vi "Data Transmit.vi"() -> ()   [LabVIEW 2021]
panel:
  in  "Message":string
  in  "Boolean":bool
  out "error out":errorcluster
  in  "error in":errorcluster
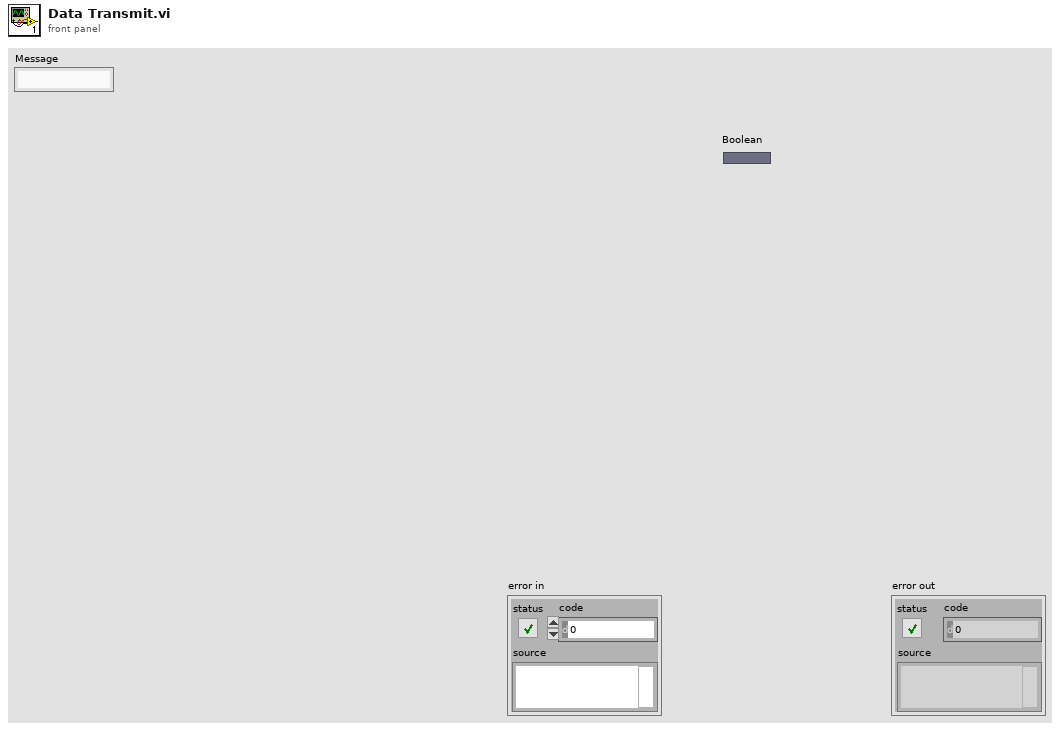
[diagram p1: front panel]
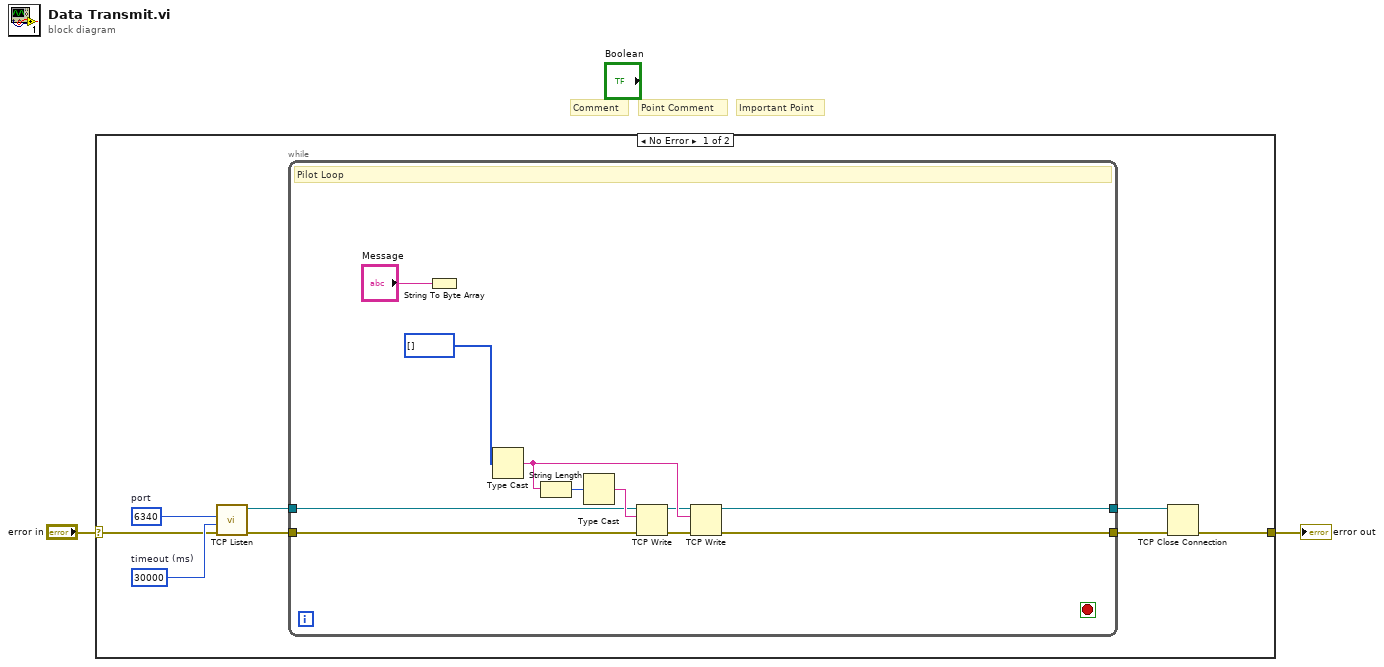
[diagram p0: block diagram]
diagram:
  # "Important Point"
  # "Point Comment"
  # "Comment"
  n1 = case shown="No Error" "error in" {
    selector: "error in" -> [w8 w22]
    tunnel: [w5 w22] -> w2
    frame No Error {
      w9 = u16 6340  # port
      w10 = 30000  # timeout (ms)
      n2 = call <vilib>:"TCP Listen.vi"("error in (no error)"=w8, "timeout ms (wait forever: -1)"=w10, "port"=w9) -> ("error out"=w7:errorcluster, "connection ID"=w4:refnum<k5>)  [unwired: 4 in, 3 out]
      n3 = while {
        tunnel: w7 -> [w14]
        tunnel: [w21] -> w6
        tunnel: w4 -> [w13]
        tunnel: [w20] -> w3
        stop <- _ stop-if-true
        # "Pilot Loop"
        n4 = String To Byte Array(string="Message") -> ()  [unwired: 1 out]
        n5 = Type Cast(x=u8[] []) -> (*(type *) &x=w19:string)  [unwired: 1 out]
        n6 = String Length(string=w19) -> (length=w17:i32)
        n7 = Type Cast(x=w17) -> (*(type *) &x=w18:string)  [unwired: 1 out]
        n8 = TCP Write(connection ID=w13, data in=w18, error in (no error)=w14) -> (connection ID out=w15:refnum<k5>, error out=w16:errorcluster)  [unwired: 2 out]
        n9 = TCP Write(connection ID=w15, data in=w19, error in (no error)=w16) -> (connection ID out=w20:refnum<k5>, error out=w21:errorcluster)  [unwired: 2 out]
      }
      n10 = TCP Close Connection(connection ID=w3, error in (no error)=w6) -> (error out=w5:errorcluster)  [unwired: 2 out]
    }
    frame Error {
    }
  }
  "error out" <- w2
